vi "measure_current_keithley-2450_python.vi"(0 "VISA resource name":refnum<visa-resource-name>="GPIB1::24::INSTR", 1 "voltage (V)":string="0", 2 "compliance (A)":string="0.1", 3 "nplc":string="0.01", 4 "settling delay (s)":string="0", 5 "error in (no error)":errorcluster) -> (14 "VISA resource name 2":refnum<visa-resource-name>="GPIB1::24::INSTR", 15 "current (A)":string, 19 "error out":errorcluster)   [LabVIEW 2016]
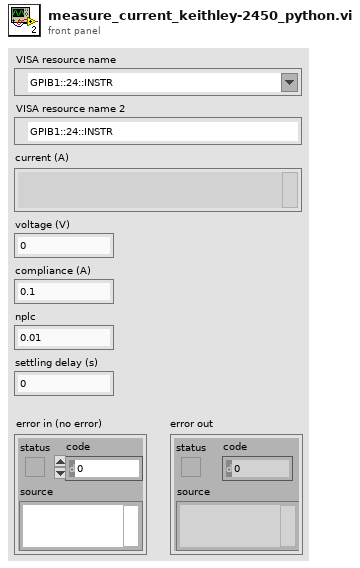
[diagram p1: front panel]
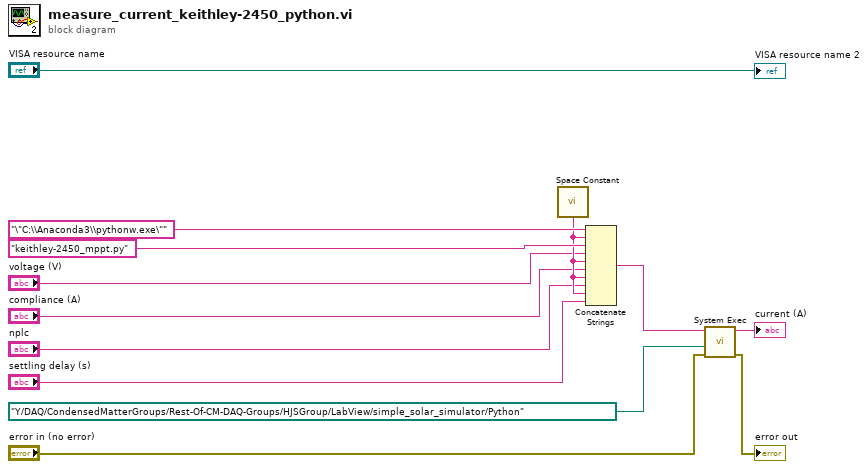
[diagram p0: block diagram]
diagram:
  n1 = call <vilib>:"Space Constant.vi"() -> ("String"=w6:string)
  n2 = Concatenate Strings("\"C:\\Anaconda3\\pythonw.exe\"" ("standard input"), w6, "keithley-2450_mppt.py" ("standard input"), "voltage (V)", w6, "compliance (A)", w6, "nplc", w6, "settling delay (s)") -> (w1:string)
  n3 = call <vilib>:"System Exec.vi"("error in (no error)"="error in (no error)", "working directory"=path "Y:/DAQ/CondensedMatterGroups/Rest-Of-CM-DAQ-Groups/HJSGroup/LabView/simple_solar_simulator/Python", "command line"=w1) -> ("error out"=→"error out":errorcluster, "standard output"=→"current (A)":string)  [unwired: 5 in, 2 out]
  "VISA resource name 2" <- "VISA resource name"
